vi "Gestione grafico.vi"(0 "Array":cluster{"X":dbl[], "Y":dbl[]}[](array[cluster]), 1 "colori grafico":T1, 2 "PLOT LEGEND":refnum<vi>, 3 "graph ref":refnum<vi>, 4 "Update annotation?":bool) -> (7 "Array out":cluster{"X":dbl[], "Y":dbl[]}[](array[cluster]))   [LabVIEW 2019]
uses:
  <vilib>/Utility/miscctls.llb/LVAnnotationListTypeDef.ctl
  <vilib>/Analysis/1siggen.llb/Ramp Pattern by Samples.vi
  <vilib>/Analysis/NI_AALPro.lvlib
  <vilib>/Analysis/NI_AALBase.lvlib
panel:
  out "Annotation List":T2
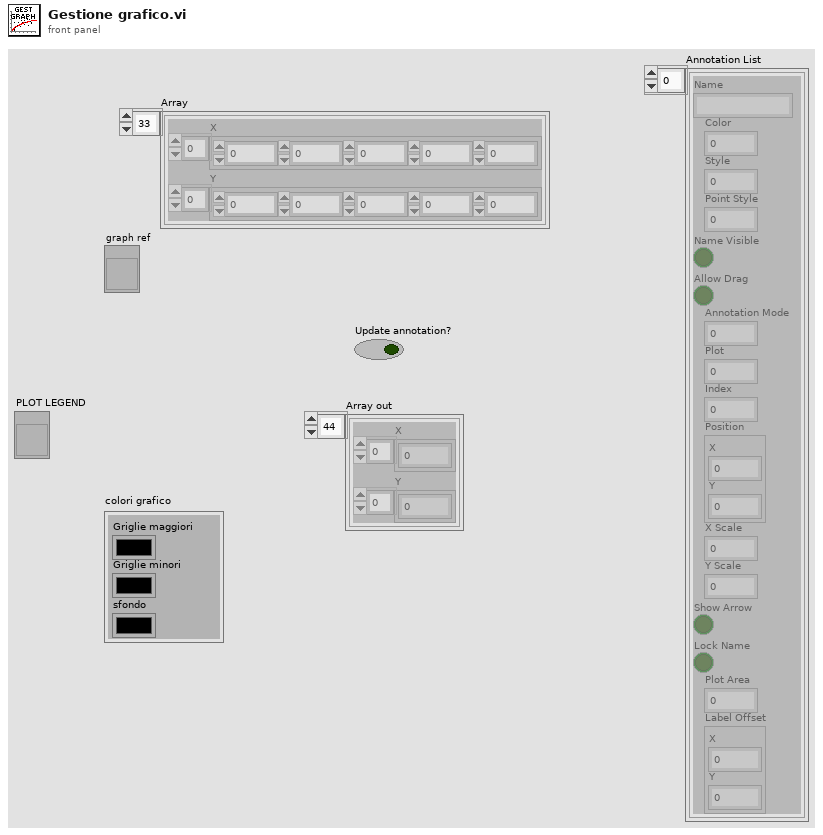
[diagram p1: front panel]
types:
  T1 = cluster{"Griglie maggiori":u32, "Griglie minori":u32, "sfondo":u32}
  T2 = typedef "LVAnnotationListTypeDef.ctl" = cluster{"Name":string, "Color":u32, "Style":u8, "Point Style":u8, "Name Visible":bool, "Allow Drag":bool, "Annotation Mode":u32, "Plot":i32, "Index":i32, "Position":cluster{"X":dbl, "Y":dbl}, "X Scale":u32, "Y Scale":u32, "Show Arrow":bool, "Lock Name":bool, "Plot Area":i32, "Label Offset":cluster{"X":dbl, "Y":dbl}}[]
  T3 = typedef "custom plot legend.ctl" = cluster{"nome plot":string, "colore":u32, "Larghezza linea":u16, "stile linea":u16, "stile punto":u16, "Visibile?":bool, "interpola?":bool, "ordine":dbl, "ScalaY":dbl, "Etichetta?":bool, "Freccia? 2":bool, "nome tab?":bool}
  T4 = cluster{"Name":string, "Color":u32, "Style":u8, "Point Style":u8, "Name Visible":bool, "Allow Drag":bool, "Annotation Mode":u32, "Plot":i32, "Index":i32, "Position":cluster{"X":i32, "Y":i32}, "X Scale":u32, "Y Scale":u32, "Show Arrow":bool, "Lock Name":bool, "Plot Area":i32, "Label Offset":cluster{"X":i32, "Y":i32}}
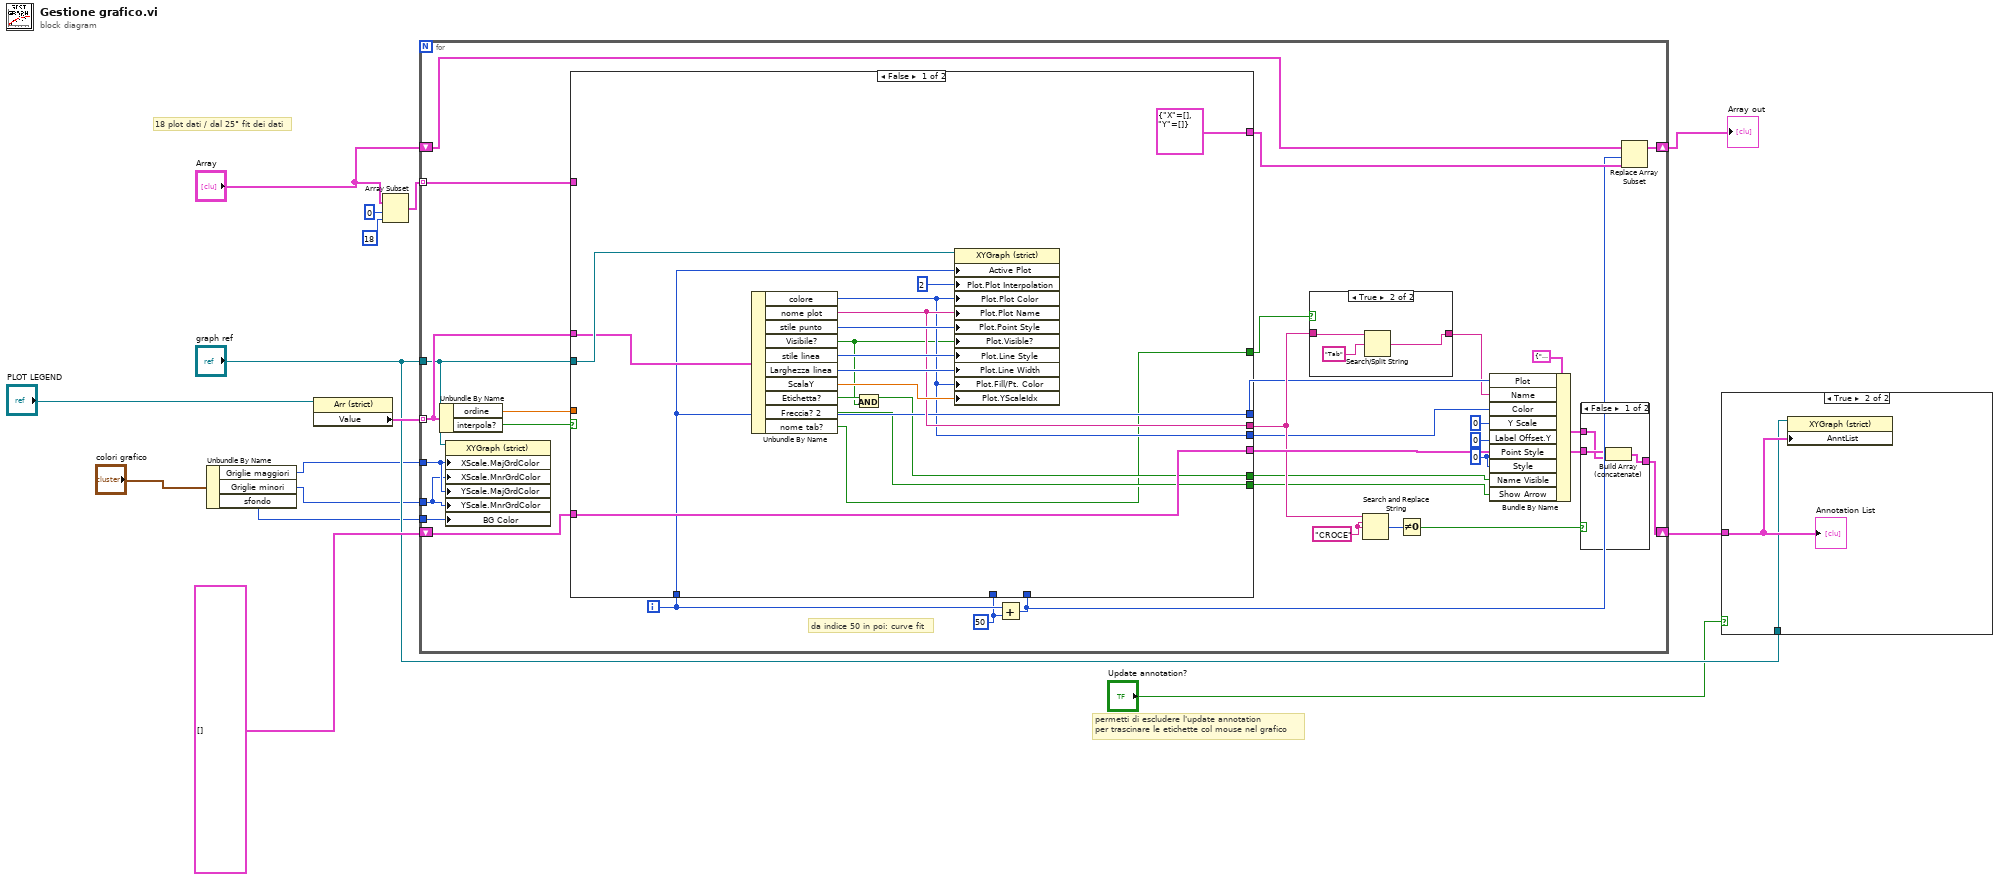
[diagram p0: block diagram]
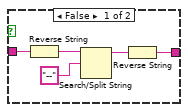
[diagram p3: hidden frame]
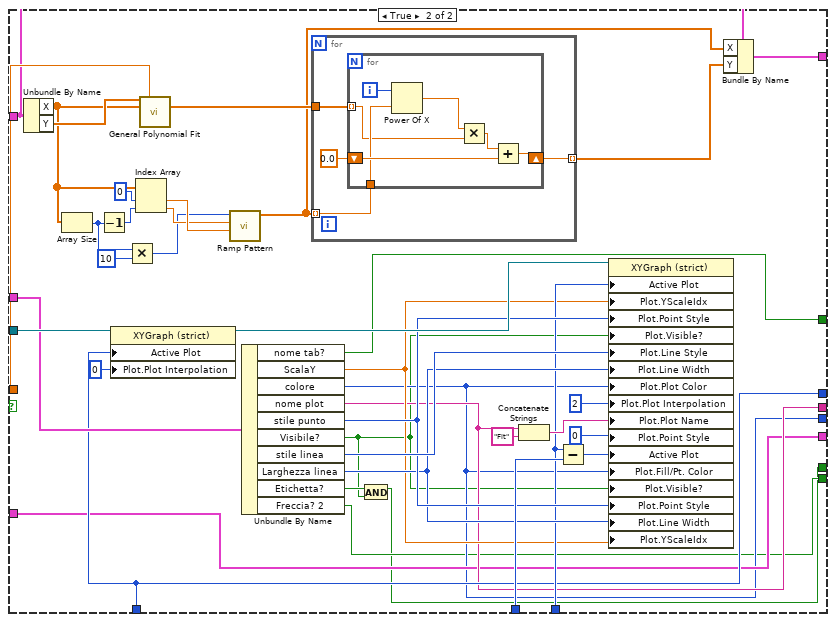
[diagram p5: hidden frame]
diagram:
  # "permetti di escludere l'update annotation\nper trascinare le etichette col mouse nel grafico"
  # "18 plot dati / dal 25° fit dei dati"
  n1 = Unbundle By Name("colori grafico") -> ("Griglie maggiori"=w5:u32, "Griglie minori"=w4:u32, "sfondo"=w2:u32)
  n2 = property class="Arr (strict)"(reference="PLOT LEGEND") -> ("Value"=w10:T3[])  [unwired: 1 in, 2 out]
  n3 = Array Subset(array="Array", index=0, length=18) -> (w12:cluster{"X":dbl[], "Y":dbl[]}[])
  n4 = for {
    tunnel: w12 -> [w47] mode=indexing
    shift-right: [w46] -> w14
    shift-left: "Array" -> [w45]
    tunnel: "graph ref" -> [w22]
    tunnel: w10 -> [w39] mode=indexing
    shift-right: [w23] -> w8
    shift-left: T2 [] ("Annotation List") -> [w37]
    tunnel: w5 -> [w21]
    tunnel: w4 -> [w20]
    tunnel: w2 -> [w19]
    i -> [w42]
    w36 = u8 0 ("Point Style")
    w31 = "CROCE" ("search string")
    w38 = 50 ("y")
    # "da indice 50 in poi: curve fit"
    n5 = Unbundle By Name(w39) -> ("ordine"=w40:dbl, "interpola?"=w41:bool)
    n6 = property class="XYGraph (strict)"(reference=w22, "XScale.MajGrdColor"=w21, "XScale.MnrGrdColor"=w20, "YScale.MajGrdColor"=w21, "YScale.MnrGrdColor"=w20, "BG Color"=w19) -> ()  [unwired: 1 in, 2 out]
    n7 = Add(x=w42, y=w38) -> (x+y=w43:i32)
    n8 = case shown="False" w41 {
      tunnel: w47 -> [_ w92]
      tunnel: [cluster{"X":dbl[], "Y":dbl[]} {"X"=[], "Y"=[]} ("QP") w103] -> w44
      tunnel: w22 -> [w75 w99]
      tunnel: w43 -> [_ w87]
      tunnel: w42 -> [w66 w85]
      tunnel: w40 -> [_ w98]
      tunnel: w39 -> [w74 w95]
      tunnel: w38 -> [_ w90]
      tunnel: w37 -> [w68 w83]
      tunnel: [w68 w83] -> w28
      tunnel: [w67 w84] -> w27
      tunnel: [w66 w85] -> w26
      tunnel: [w62 w79] -> w25
      tunnel: [w65 w82] -> w24
      tunnel: [w63 w80] -> w18
      tunnel: [w60 w77] -> w16
      frame False {
        n9 = Unbundle By Name(w74) -> ("colore"=w65:u32, "nome plot"=w67:string, "stile punto"=w73:u16, "Visibile?"=w61:bool, "stile linea"=w72:u16, "Larghezza linea"=w71:u16, "ScalaY"=w69:dbl, "Etichetta?"=w64:bool, "Freccia? 2"=w63:bool, "nome tab?"=w60:bool)
        n10 = And(x=w64, y=w61) -> (x .and. y?=w62:bool)
        n11 = property class="XYGraph (strict)"(reference=w75, "Active Plot"=w66, "Plot.Plot Interpolation"=u8 2, "Plot.Plot Color"=w65, "Plot.Plot Name"=w67, "Plot.Point Style"=w73, "Plot.Visible?"=w61, "Plot.Line Style"=w72, "Plot.Line Width"=w71, "Plot.Fill/Pt. Color"=w65, "Plot.YScaleIdx"=w69) -> ()  [unwired: 1 in, 2 out]
      }
      frame True {
        n12 = Unbundle By Name(w92) -> ("X"=w104:dbl[], "Y"=w105:dbl[])
        n13 = Array Size(array=w104) -> (size(s)=w111:i32)
        n14 = Decrement(x=w111) -> (x-1=w114:i32)
        n15 = property class="XYGraph (strict)"(reference=w99, "Active Plot"=w85, "Plot.Plot Interpolation"=u8 0) -> (reference out=w93:refnum<vi>)  [unwired: 1 in, 1 out]
        n16 = Multiply(x=w111, y=10) -> (x*y=w109:i32)
        n17 = Index Array(array=w104, index #1=0 ("index"), index #2=w114) -> (element #1=w113:dbl, element #2=w112:dbl)
        n18 = call <vilib>:"General Polynomial Fit.vi"("Y"=w105, "polynomial order"=w98, "X"=w104) -> ("Polynomial Coefficients"=w108:dbl[])  [unwired: 9 in, 3 out]
        n19 = call-poly <vilib>:"Ramp Pattern.vi"("start"=w113, "end"=w112, "samples"=w109) -> ("Ramp Pattern"=w107:dbl[])  [unwired: 7 in, 1 out]
        n20 = Unbundle By Name(w95) -> ("nome tab?"=w77:bool, "ScalaY"=w86:dbl, "colore"=w82:u32, "nome plot"=w84:string, "stile punto"=w89:u16, "Visibile?"=w78:bool, "stile linea"=w94:u16, "Larghezza linea"=w88:u16, "Etichetta?"=w81:bool, "Freccia? 2"=w80:bool)
        n21 = for {
          tunnel: w108 -> [w119]
          tunnel: [w117] -> w106 mode=indexing
          tunnel: w107 -> [w116] mode=indexing
          n22 = for {
            tunnel: w119 -> [w120] mode=indexing
            tunnel: w116 -> [w121]
            shift-right: [w124] -> w117
            shift-left: 0.0 -> [w123]
            i -> [w122]
            n23 = Power Of X(1:w121, 2:w122) -> (0:w126:dbl)
            n24 = Multiply(x=w126, y=w120) -> (x*y=w125:dbl)
            n25 = Add(x=w125, y=w123) -> (x+y=w124:dbl)
          }
        }
        n26 = And(x=w81, y=w78) -> (x .and. y?=w79:bool)
        n27 = Concatenate Strings(w84, "Fit" ("string")) -> (w102:string)
        n28 = Subtract(x=w87, y=w90) -> (x-y=w91:i32)
        n29 = property class="XYGraph (strict)"(reference=w93, "Active Plot"=w87, "Plot.YScaleIdx"=w86, "Plot.Point Style"=w89, "Plot.Visible?"=w78, "Plot.Line Style"=w94, "Plot.Line Width"=w88, "Plot.Plot Color"=w82, "Plot.Plot Interpolation"=u8 2, "Plot.Plot Name"=w102, "Plot.Point Style"=u8 0, "Active Plot"=w91, "Plot.Fill/Pt. Color"=w82, "Plot.Visible?"=w78, "Plot.Point Style"=w89, "Plot.Line Width"=w88, "Plot.YScaleIdx"=w86) -> ()  [unwired: 1 in, 2 out]
        n30 = Bundle By Name(cluster=w92, "X"=w107, "Y"=w106) -> (w103:cluster{"X":dbl[], "Y":dbl[]})
      }
    }
    n31 = case shown="True" w16 {
      tunnel: w27 -> [w49 w54]
      tunnel: [w48 w53] -> w17
      frame False {
        n32 = Reverse String(1:w49) -> (0:w50:string)
        n33 = Search/Split String(string=w50, search string/char (-)="--") -> (substring before match=w52:string)  [unwired: 1 in, 2 out]
        n34 = Reverse String(1:w52) -> (0:w48:string)
      }
      frame True {
        n35 = Search/Split String(string=w54, search string/char (-)="Tab") -> (match + rest of string=w53:string)  [unwired: 1 in, 2 out]
      }
    }
    n36 = Search and Replace String(input string=w27, search string=w31, replace string=w31) -> (number of replacements=w32:i32)  [unwired: 5 in, 3 out]
    n37 = Not Equal To 0?(x=w32) -> (x != 0?=w33:bool)
    n38 = Bundle By Name(cluster=T4 {"Name"="0", "Color"=589961, "Style"=4, "Point Style"=13, "Name Visible"=TRUE, "Allow Drag"=TRUE, "Annotation Mode"=1, "Plot"=1, "Index"=4, "Position"={"X"=0, "Y"=0}, "X Scale"=0, "Y Scale"=1, "Show Arrow"=FALSE, "Lock Name"=FALSE, "Plot Area"=0, "Label Offset"={"X"=0, "Y"=0}}, "Plot"=w26, "Name"=w17, "Color"=w24, "Y Scale"=u32 0, "Label Offset.Y"=0, "Point Style"=w36, "Style"=w36, "Name Visible"=w25, "Show Arrow"=w18) -> (w30:T4)
    n39 = case shown="False" w33 {
      tunnel: w28 -> [w58 w59]
      tunnel: w30 -> [w57 _]
      tunnel: [w56 w59] -> w23
      frame False {
        n40 = Build Array (concatenate)(w58, w57) -> (w56:T2)
      }
      frame True {
      }
    }
    n41 = Replace Array Subset(array=w45, new element=w44, index=w43) -> (w46:cluster{"X":dbl[], "Y":dbl[]}[])
  }
  "Array out" <- w14
  n42 = case shown="True" "Update annotation?" {
    tunnel: w8 -> [_ w128]
    tunnel: "graph ref" -> [_ w127]
    frame False {
    }
    frame True {
      n43 = property class="XYGraph (strict)"(reference=w127, "AnntList"=w128) -> ()  [unwired: 1 in, 2 out]
      "Annotation List" <- w128
    }
  }
